vi "Stop Core.vi"(10 "final error code":i32, 11 "InferenceTCP in":refnum<class "InferenceTCP.lvclass">) -> (3 "InferenceTCP out":refnum<class "InferenceTCP.lvclass">)   [LabVIEW 2019, in "InferenceTCP.lvlib" / "InferenceTCP.lvclass"]
doc: "(<B>Filename</B>: Actor Framework.lvlib:Actor.lvclass:Stop Core.vi)\n\nDefines what the actor does before it stops. Use the <B>final error code</B> input to determine whether the actor shut down in response to an error.\n\nBy default, this method passes the Stop message along to all auto-stop nested actors. A descendant class may override this method to define additional behavior, such as shutting down any processes the actor initiated in its override of the Actor Core method."
uses:
  InferenceTCP.lvclass
  InferenceTCP.lvclass/InferenceTCP.ctl
  Inference/Inference/Inference.lvclass
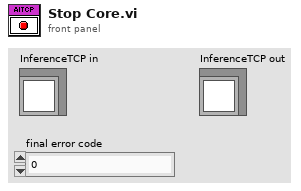
[diagram p1: front panel]
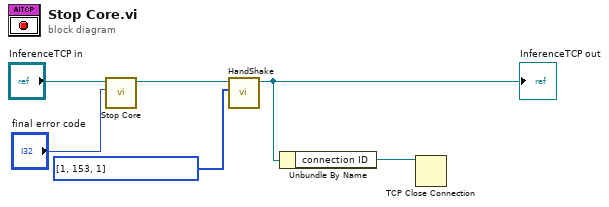
[diagram p0: block diagram]
diagram:
  n1 = call-parent "Stop Core.vi"("final error code"="final error code", "Actor in"="InferenceTCP in") -> ("Actor out"=w3:refnum<class "InferenceTCP.lvclass">)  [unwired: 9 in]
  n2 = call "HandShake.vi"("Data In"=u8[] [1, 153, 1], "InferenceTCP in"=w3) -> ("InferenceTCP out"=w2:refnum<class "InferenceTCP.lvclass">)  [unwired: 7 in, 2 out]
  "InferenceTCP out" <- w2
  n3 = Unbundle By Name(w2) -> ("connection ID"=w1:refnum<k5>)
  n4 = TCP Close Connection(connection ID=w1) -> ()  [unwired: 2 in, 2 out]
